vi "Teardown.vi"(6 "Error":errorcluster, 7 "ConcreteActor":refnum<class "ConcreteActor.lvclass">, 10 "TeardownLocation":T1, 11 "UnheardMessages":refnum<class "Message.lvclass">[](array[class])) -> (5 "ConcreteActor":refnum<class "ConcreteActor.lvclass">)   [LabVIEW 2020, in "_Template.lvlib" / "ActorTemplate.lvlib" / "{{Name}}.lvlib" / "ConcreteActor.lvclass"]
uses:
  ConcreteActor.lvclass
  jettl/jettl/Message/Message.lvclass
  ConcreteActor.lvclass/ConcreteActor.ctl
  jettl/jettl/Actor/Actor.lvclass
  jettl/jettl/TeardownLocation.ctl
  jettl/jettl/jettl.lvlib
panel:
  # "This front panel should not be manipulated."
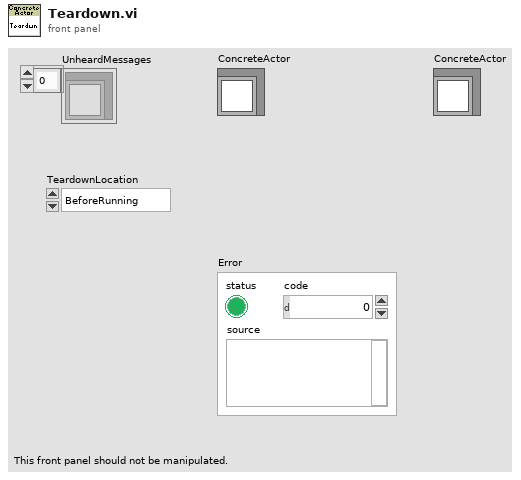
[diagram p1: front panel]
types:
  T1 = typedef "jettl.lvlib/TeardownLocation.ctl" = enum16{"BeforeRunning", "AfterRunning"}
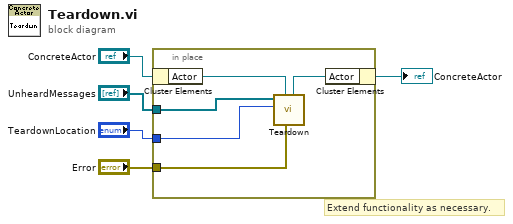
[diagram p0: block diagram]
diagram:
  # "Extend functionality as necessary."
  n1 = in-place {
    in-place-border: "UnheardMessages" -> [w8]
    in-place-border: "TeardownLocation" -> [w7]
    in-place-border: "Error" -> [w6]
    n2 = in-place-cluster #1("ConcreteActor") -> ("Actor"=w10:refnum<class "Actor.lvclass">)
    n3 = call-dynamic "Teardown.vi"("Error"=w6, "Actor"=w10, "TeardownLocation"=w7, "UnheardMessages"=w8) -> ("Actor"=w9:refnum<class "Actor.lvclass">)  [unwired: 7 in]
    n4 = in-place-cluster #1("Actor"=w9) -> (→"ConcreteActor":refnum<class "ConcreteActor.lvclass">)
  }
